vi "Write Index Visible.vi"(8 "error in (no error)":errorcluster, 10 "IndexVis":bool, 11 "Array.lvclass in":refnum<class "Array.lvclass">) -> (0 "error out":errorcluster, 3 "Array.lvclass out":refnum<class "Array.lvclass">)   [LabVIEW 2015, in "Array.lvclass"]
uses:
  Array.lvclass
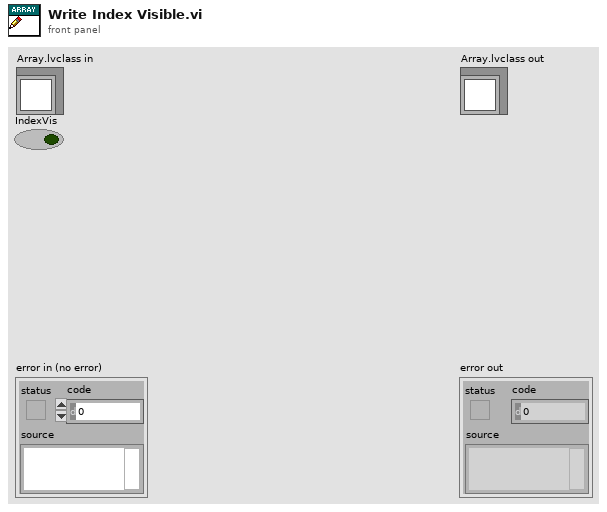
[diagram p1: front panel]
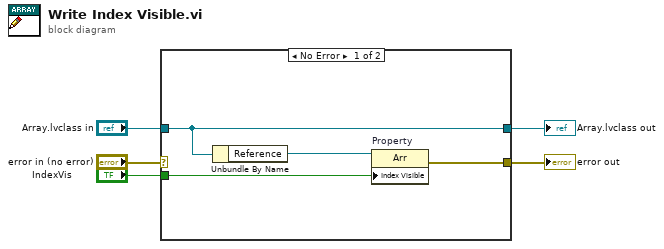
[diagram p0: block diagram]
diagram:
  n1 = case shown="No Error" "error in (no error)" {
    selector: "error in (no error)" -> [_ w11]
    tunnel: [w9 w11] -> w4
    tunnel: [w7 w10] -> w2
    tunnel: "Array.lvclass in" -> [w7 w10]
    tunnel: "IndexVis" -> [w8 _]
    frame No Error {
      n2 = Unbundle By Name(w7) -> ("Reference"=w6:refnum<vi>)
      n3 = property on="Property" class="Arr"(reference=w6, "Index Visible"=w8) -> (error out=w9:errorcluster)  [unwired: 1 in, 1 out]
    }
    frame Error {
    }
  }
  "error out" <- w4
  "Array.lvclass out" <- w2
